vi "Axial Waveform Scan Done.vi"(8 "error in (no error)":errorcluster, 11 "Model in":refnum<class "Model.lvclass">) -> (0 "error out":errorcluster, 2 "Done":bool, 3 "Model out":refnum<class "Model.lvclass">)   [LabVIEW 2015, in "Model.lvclass"]
uses:
  Model.lvclass
  Model.lvclass/Model.ctl
  Waveforms/Waveform/Waveform.lvclass
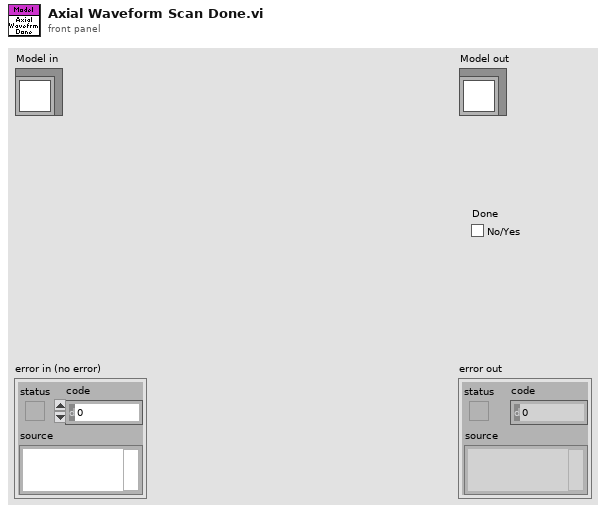
[diagram p1: front panel]
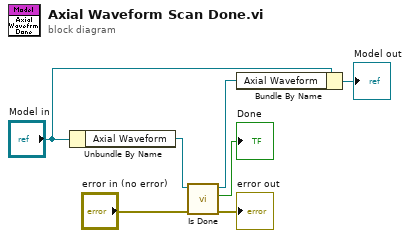
[diagram p0: block diagram]
diagram:
  n1 = Unbundle By Name("Model in") -> ("Axial Waveform"=w7:refnum<class "Waveform.lvclass">)
  n2 = call-dynamic "Is Done.vi"("error in (no error)"="error in (no error)", "Waveform in"=w7) -> ("error out"=→"error out":errorcluster, "Is Done"=→"Done":bool, "Waveform out"=w1:refnum<class "Waveform.lvclass">)  [unwired: 7 in]
  n3 = Bundle By Name(cluster="Model in", "Axial Waveform"=w1) -> (→"Model out":refnum<class "Model.lvclass">)
